vi "Register Events.vi"(0 "reference in":refnum<class "HPS-17000-PowerModule.lvclass">, 11 "Error In":errorcluster) -> (4 "reference out":refnum<class "HPS-17000-PowerModule.lvclass">, 15 "Error Out":errorcluster)   [LabVIEW 2023, in "HPS-17000-PowerModule.lvlib" / "HPS-17000-PowerModule.lvclass"]
uses:
  HPS-17000-PowerModule.lvclass
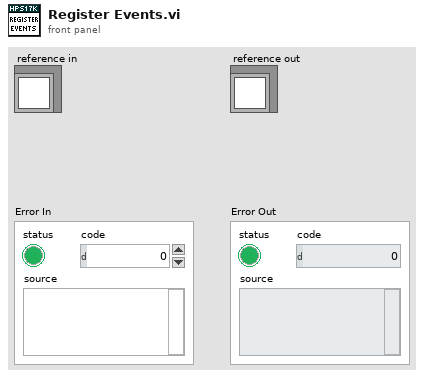
[diagram p1: front panel]
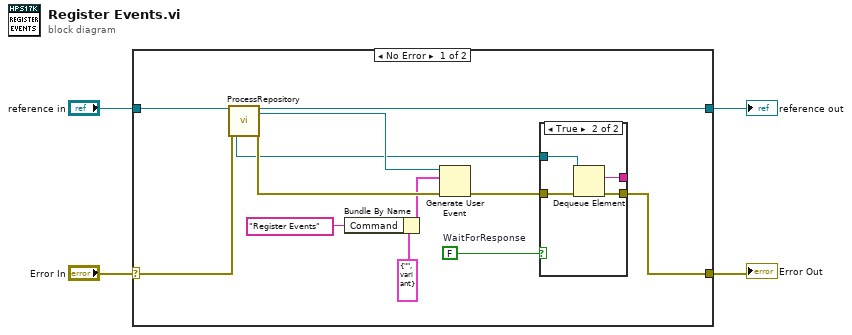
[diagram p0: block diagram]
diagram:
  n1 = case shown="No Error" "Error In" {
    selector: "Error In" -> [w16 w23]
    tunnel: [w9 w23] -> w3
    tunnel: [w14 w22] -> w1
    tunnel: "reference in" -> [w15 w22]
    frame No Error {
      w12 = FALSE  # WaitForResponse
      n2 = call "ProcessRepository.vi"("reference in"=w15, "Error In"=w16) -> ("QueueFromProcess"=w6:refnum<queue>, "reference out"=w14:refnum<class "HPS-17000-PowerModule.lvclass">, "EventsToProcess"=w13:refnum<user-event>, "Error Out"=w10:errorcluster)  [unwired: 10 in, 4 out]
      n3 = Bundle By Name(cluster=cluster{"Command":string, "Data":variant} {"Command"="", "Data"=variant} ("MessageToProcess"), "Command"="Register Events") -> (w7:cluster{"Command":string, "Data":variant})
      n4 = Generate User Event(user event=w13, event data cluster=w7, error in=w10) -> (error out=w11:errorcluster)  [unwired: 1 in, 1 out]
      n5 = case shown="True" w12 {
        tunnel: w11 -> [w17 w21]
        tunnel: [_ w20] -> _
        tunnel: [w17 w19] -> w9
        tunnel: w6 -> [_ w18]
        frame False {
        }
        frame True {
          n6 = Dequeue Element(queue=w18, error in (no error)=w21) -> (element=w20:string, error out=w19:errorcluster)  [unwired: 1 in, 2 out]
        }
      }
    }
    frame Error {
    }
  }
  "Error Out" <- w3
  "reference out" <- w1
